vi "Make Sender.vi"(8 "error in (no error)":errorcluster, 11 "Message Scripter in":refnum<class "Message Scripter.lvclass">) -> (0 "error out":errorcluster, 3 "Message Scripter out":refnum<class "Message Scripter.lvclass">)   [LabVIEW 2020, in "Message Maker.lvlib" / "Message Scripter.lvclass"]
uses:
  Message Scripter.lvclass
  Send Builder/Send Builder.lvclass
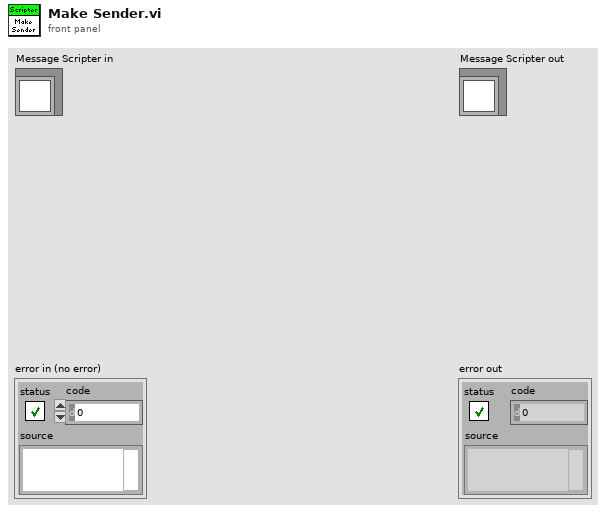
[diagram p1: front panel]
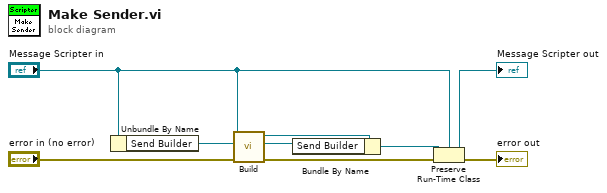
[diagram p0: block diagram]
diagram:
  n1 = Unbundle By Name("Message Scripter in") -> ("Send Builder"=w9:refnum<class "Send Builder.lvclass">)
  n2 = call-dynamic "Build.vi"("error in (no error)"="error in (no error)", "Send Builder in"=w9, "Message Maker in"="Message Scripter in") -> ("error out"=w7:errorcluster, "Send Builder out"=w8:refnum<class "Send Builder.lvclass">, "Message Maker out"=w2:refnum<class "Message Scripter.lvclass">)  [unwired: 6 in]
  n3 = Bundle By Name(cluster=w2, "Send Builder"=w8) -> (w1:refnum<class "Message Scripter.lvclass">)
  n4 = Preserve Run-Time Class(object in=w1, error in=w7, 2:"Message Scripter in") -> (object out=→"Message Scripter out":refnum<class "Message Scripter.lvclass">, error out=→"error out":errorcluster)
